vi "Begin.vi"() -> (0 "error out":errorcluster)   [LabVIEW 2012]
doc: "Called before other user functions, this VI is expected to open initial I/O refnums, load in file data, and do all program initialization. Notice that the <B>error out</B> terminal is simply used for data flow. Wiring it to other structures or subVIs ensures that this VI runs first."
uses:
  <vilib>/Rock Robotics/WPI/Joystick/WPI_JoystickDeviceEnum.ctl
  <vilib>/Rock Robotics/SystemInterfaces/Typedef/FPGA_TypedefDigitalModule.ctl
  <vilib>/Rock Robotics/SystemInterfaces/DIO/FPGA_DIOPWMChannel.ctl
  <vilib>/Rock Robotics/WPI/SafetyOutput/WPI_SafetyOutputConfigMenu.ctl
  <vilib>/Rock Robotics/WPI/CAN/Jaguar/SubVIs/WPI_CANJaguar_ControlMode.ctl
  <vilib>/Rock Robotics/WPI/CAN/Jaguar/SubVIs/WPI_CANJaguar_SpeedReference.ctl
  <vilib>/Rock Robotics/WPI/CAN/Jaguar/SubVIs/WPI_CANJaguar_BrakeCoastMode.ctl
  Robot Global Data.vi
  <vilib>/Rock Robotics/WPI/MotorControl/WPI_MotorControlOpen Victor.vi
  <vilib>/Rock Robotics/WPI/MotorControl/WPI_MotorControlOpenCANJaguar.vi
  <vilib>/Rock Robotics/WPI/RobotDrive/WPI_RobotDriveOpen2MotorWithCANJaguar.vi
  <vilib>/Rock Robotics/SystemInterfaces/AI/FPGA_AIGyroChannel.ctl
  <vilib>/Rock Robotics/SystemInterfaces/Typedef/FPGA_TypedefAnalogModuleForGyro.ctl
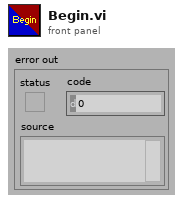
[diagram p1: front panel]
types:
  T1 = typedef "WPI_SafetyOutputConfigMenu.ctl" = enum16{"Enable", "Disable"}
  T2 = typedef "FPGA_DIOPWMChannel.ctl" = enum8{"PWM 1", "PWM 2", "PWM 3", "PWM 4", "PWM 5", "PWM 6", "PWM 7", "PWM 8", "PWM 9", "PWM 10", "Invalid"}
  T3 = typedef "FPGA_TypedefDigitalModule.ctl" = enum16{"Digital Module 1", "Digital Module 2"}
  T4 = typedef "WPI_JoystickDeviceEnum.ctl" = enum16{"USB 1", "USB 2", "USB 3", "USB 4", "Kinect 1", "Kinect 2"}
  T5 = typedef "WPI_MotorControlDeviceRef.ctl" = cluster{"DeviceStatus":errorcluster, "Type":enum16{"PWM", "CAN"}, "PWM":cluster{"Digital Module":T3, "PWM Channel":T2, "DeadBand":T6}, "CAN":cluster{"Device Number":u8, "Control Mode":T7, "Semaphore":T8, "Max Vout":dbl}, "Invert":bool, "TransformRef":T9, "InvTransformRef":T9}
  T6 = typedef "WPI_PWMDeadband.ctl" = cluster{"Name":string, "maxPositivePwm":i32, "minPositivePwm":i32, "centerPwm":i32, "maxNegativePwm":i32, "minNegativePwm":i32, "angularRange":u16}
  T7 = typedef "WPI_CANJaguar_ControlMode.ctl" = enum8{"Percent VBus", "Current", "Speed", "Position", "Voltage"}
  T8 = typedef "Semaphore RefNum" = refnum<k1>
  T9 = typedef "WPI_PWMTransform_ConPane.ctl" = refnum<vi>
  T10 = typedef "WPI_ServoDeviceRef.ctl" = cluster{"DeviceStatus":errorcluster, "Digital Module":T3, "PWM Channel":T2, "DeadBand":T6}
  T11 = typedef "WPI_RobotDriveDevRef.ctl" = cluster{"DevStatus":errorcluster, "Motors[]":T5[], "Square Inputs":bool, "Max Output":dbl, "Isochronous":bool}
  T12 = typedef "WPI_CANJaguar_BrakeCoastMode.ctl" = enum8{"Jumper", "Brake", "Coast"}
  T13 = typedef "WPI_CANJaguar_SpeedReference.ctl" = u8
  T14 = typedef "WPI_JoystickDevRef.ctl" = cluster{"Device":T4}
  T15 = typedef "FPGA_TypedefAnalogModuleForGyro.ctl" = enum16{"Analog Module 1"}
  T16 = typedef "FPGA_AIGyroChannel.ctl" = enum8{"AI 1", "AI 2", "Invalid"}
  T17 = typedef "WPI_GyroDevRef.ctl" = cluster{"DevStatus":errorcluster, "Analog Module":T18, "Analog Channel":T19, "Offset":dbl, "Gain (VoltsPerDegree/Second)":dbl}
  T18 = typedef "FPGA_TypedefAnalogModule.ctl" = enum16{"Analog Module 1", "Analog Module 2"}
  T19 = typedef "FPGA_AIChannel.ctl" = enum8{"AI 1", "AI 2", "AI 3", "AI 4", "AI 5", "AI 6", "AI 7", "AI 8", "Invalid"}
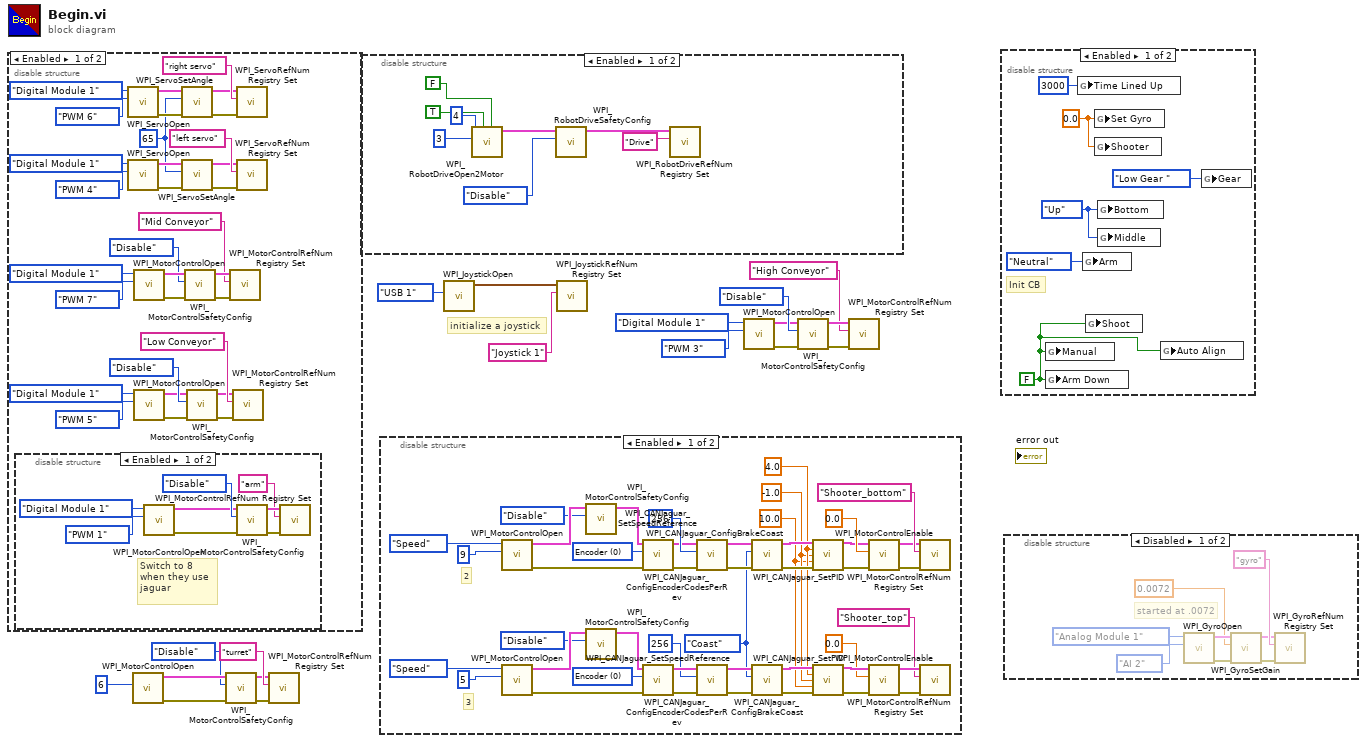
[diagram p0: block diagram]
diagram:
  # "initialize a joystick"
  n1 = disable-structure shown="Enabled" {
    frame Enabled {
      w19 = 65 ("Angle")
      n2 = disable-structure shown="Enabled" {
        frame Enabled {
          # "Switch to 8\nwhen they use\njaguar"
          n3 = call-poly <vilib>:"WPI_MotorControlOpen.vi"("PWM Channel"=FPGA_DIOPWMChannel."PWM 1", "Digital Module (Module 1)"=FPGA_TypedefDigitalModule."Digital Module 1") -> ("error out"=w53:errorcluster, "MotorControlDeviceRef"=w54:T5)  [unwired: 8 in]
          n4 = call <vilib>:"WPI_MotorControlSafetyConfig.vi"("error in (no error)"=w53, "mode"=WPI_SafetyOutputConfigMenu."Disable", "MotorControlDevRef"=w54) -> ("error out"=w51:errorcluster, "MotorControlDevRef"=w52:T5)  [unwired: 7 in]
          n5 = call <vilib>:"WPI_MotorControlRefNum Registry Set.vi"("error in (no error)"=w51, "refnum name"="arm", "MotorControlDevRef"=w52) -> ()  [unwired: 7 in, 2 out]
        }
        frame Disabled {
        }
      }
      n6 = call <vilib>:"WPI_ServoOpen.vi"("PWM Channel"=FPGA_DIOPWMChannel."PWM 6", "Digital Module (Module 1)"=FPGA_TypedefDigitalModule."Digital Module 1") -> ("error out"=w25:errorcluster, "ServoDeviceRef"=w27:T10)  [unwired: 8 in]
      n7 = call <vilib>:"WPI_ServoOpen.vi"("PWM Channel"=FPGA_DIOPWMChannel."PWM 4", "Digital Module (Module 1)"=FPGA_TypedefDigitalModule."Digital Module 1") -> ("error out"=w21:errorcluster, "ServoDeviceRef"=w23:T10)  [unwired: 8 in]
      n8 = call-poly <vilib>:"WPI_MotorControlOpen.vi"("PWM Channel"=FPGA_DIOPWMChannel."PWM 7", "Digital Module (Module 1)"=FPGA_TypedefDigitalModule."Digital Module 1") -> ("error out"=w41:errorcluster, "MotorControlDeviceRef"=w40:T5)  [unwired: 8 in]
      n9 = call-poly <vilib>:"WPI_MotorControlOpen.vi"("PWM Channel"=FPGA_DIOPWMChannel."PWM 5", "Digital Module (Module 1)"=FPGA_TypedefDigitalModule."Digital Module 1") -> ("error out"=w31:errorcluster, "MotorControlDeviceRef"=w32:T5)  [unwired: 8 in]
      n10 = call <vilib>:"WPI_ServoSetAngle.vi"("error in (no error)"=w25, "Angle"=w19, "ServoDeviceRef"=w27) -> ("error out"=w24:errorcluster, "ServoDeviceRef"=w26:T10)  [unwired: 7 in]
      n11 = call <vilib>:"WPI_ServoSetAngle.vi"("error in (no error)"=w21, "Angle"=w19, "ServoDeviceRef"=w23) -> ("error out"=w20:errorcluster, "ServoDeviceRef"=w22:T10)  [unwired: 7 in]
      n12 = call <vilib>:"WPI_MotorControlSafetyConfig.vi"("error in (no error)"=w41, "mode"=WPI_SafetyOutputConfigMenu."Disable", "MotorControlDevRef"=w40) -> ("error out"=w43:errorcluster, "MotorControlDevRef"=w42:T5)  [unwired: 7 in]
      n13 = call <vilib>:"WPI_MotorControlSafetyConfig.vi"("error in (no error)"=w31, "mode"=WPI_SafetyOutputConfigMenu."Disable", "MotorControlDevRef"=w32) -> ("error out"=w29:errorcluster, "MotorControlDevRef"=w30:T5)  [unwired: 7 in]
      n14 = call <vilib>:"WPI_MotorControlRefNum Registry Set.vi"("error in (no error)"=w43, "refnum name"="Mid Conveyor", "MotorControlDevRef"=w42) -> ()  [unwired: 7 in, 2 out]
      n15 = call <vilib>:"WPI_MotorControlRefNum Registry Set.vi"("error in (no error)"=w29, "refnum name"="Low Conveyor", "MotorControlDevRef"=w30) -> ()  [unwired: 7 in, 2 out]
      n16 = call <vilib>:"WPI_ServoRefNum Registry Set.vi"("error in (no error)"=w24, "refnum name"="right servo", "ServoDeviceRef"=w26) -> ()  [unwired: 7 in, 2 out]
      n17 = call <vilib>:"WPI_ServoRefNum Registry Set.vi"("error in (no error)"=w20, "refnum name"="left servo", "ServoDeviceRef"=w22) -> ()  [unwired: 7 in, 2 out]
    }
    frame Disabled {
    }
  }
  n18 = call-poly <vilib>:"WPI_MotorControlOpen.vi"("Device Number"=u8 6) -> ("error out"=w4:errorcluster, "MotorControlDeviceRef"=w3:T5)  [unwired: 9 in]
  n19 = call <vilib>:"WPI_MotorControlSafetyConfig.vi"("error in (no error)"=w4, "mode"=WPI_SafetyOutputConfigMenu."Disable", "MotorControlDevRef"=w3) -> ("error out"=w6:errorcluster, "MotorControlDevRef"=w5:T5)  [unwired: 7 in]
  n20 = call <vilib>:"WPI_MotorControlRefNum Registry Set.vi"("error in (no error)"=w6, "refnum name"="turret", "MotorControlDevRef"=w5) -> ()  [unwired: 7 in, 2 out]
  n21 = disable-structure shown="Enabled" {
    frame Enabled {
      n22 = call-poly <vilib>:"WPI_RobotDriveOpen2Motor.vi"("Right Motor Inverted"=FALSE, "Left Motor Inverted"=TRUE, "Right Motor"=u8 3, "Left Motor"=u8 4) -> ("RobotDriveDevRef"=w62:T11)  [unwired: 6 in, 1 out]
      n23 = call <vilib>:"WPI_RobotDriveSafetyConfig.vi"("mode"=WPI_SafetyOutputConfigMenu."Disable", "RobotDriveDevRef"=w62) -> ("RobotDriveDevRef"=w61:T11)  [unwired: 8 in, 1 out]
      n24 = call <vilib>:"WPI_RobotDriveRefNum Registry Set.vi"("refnum name"="Drive", "RobotDriveDevRef"=w61) -> ()  [unwired: 8 in, 2 out]
    }
    frame Disabled {
    }
  }
  n25 = disable-structure shown="Enabled" {
    frame Enabled {
      w75 = WPI_CANJaguar_BrakeCoastMode."Coast" ("Brake / Coast Mode")
      w66 = 10.0 ("D")
      w67 = -1.0 ("I")
      w68 = 4.0 ("P")
      w87 = T13 0 items=["Encoder"=0, "Inv Encoder"=2, "Quad Encoder"=3, "None"=255] ("Speed Reference")
      w104 = T13 0 items=["Encoder"=0, "Inv Encoder"=2, "Quad Encoder"=3, "None"=255] ("Speed Reference")
      # "2"
      # "3"
      n26 = call-poly <vilib>:"WPI_MotorControlOpen.vi"("Device Number"=u8 9, "Control Mode"=WPI_CANJaguar_ControlMode."Speed") -> ("error out"=w86:errorcluster, "MotorControlDeviceRef"=w85:T5)  [unwired: 8 in]
      n27 = call-poly <vilib>:"WPI_MotorControlOpen.vi"("Device Number"=u8 5, "Control Mode"=WPI_CANJaguar_ControlMode."Speed") -> ("error out"=w105:errorcluster, "MotorControlDeviceRef"=w106:T5)  [unwired: 8 in]
      n28 = call <vilib>:"WPI_MotorControlSafetyConfig.vi"("mode"=WPI_SafetyOutputConfigMenu."Disable", "MotorControlDevRef"=w85) -> ("MotorControlDevRef"=w72:T5)  [unwired: 8 in, 1 out]
      n29 = call <vilib>:"WPI_MotorControlSafetyConfig.vi"("mode"=WPI_SafetyOutputConfigMenu."Disable", "MotorControlDevRef"=w106) -> ("MotorControlDevRef"=w70:T5)  [unwired: 8 in, 1 out]
      n30 = call <vilib>:"WPI_CANJaguar_SetSpeedReference.vi"("error in (no error)"=w86, "Speed Reference"=w87, "CAN Jaguar Ref"=w72) -> ("error out"=w89:errorcluster, "CAN Jaguar Ref Out"=w84:T5)  [unwired: 7 in]
      n31 = call <vilib>:"WPI_CANJaguar_SetSpeedReference.vi"("error in (no error)"=w105, "Speed Reference"=w104, "CAN Jaguar Ref"=w70) -> ("error out"=w102:errorcluster, "CAN Jaguar Ref Out"=w107:T5)  [unwired: 7 in]
      n32 = call <vilib>:"WPI_CANJaguar_ConfigEncoderCodesPerRev.vi"("error in (no error)"=w89, "Encoder Codes Per Rev"=u16 256, "CAN Jaguar Ref"=w84) -> ("error out"=w76:errorcluster, "CAN Jaguar Ref Out"=w77:T5)  [unwired: 7 in]
      n33 = call <vilib>:"WPI_CANJaguar_ConfigEncoderCodesPerRev.vi"("error in (no error)"=w102, "Encoder Codes Per Rev"=u16 256, "CAN Jaguar Ref"=w107) -> ("error out"=w80:errorcluster, "CAN Jaguar Ref Out"=w81:T5)  [unwired: 7 in]
      n34 = call <vilib>:"WPI_CANJaguar_ConfigBrakeCoast.vi"("error in (no error)"=w76, "Brake / Coast Mode"=w75, "CAN Jaguar Ref"=w77) -> ("error out"=w73:errorcluster, "CAN Jaguar Ref Out"=w74:T5)  [unwired: 7 in]
      n35 = call <vilib>:"WPI_CANJaguar_ConfigBrakeCoast.vi"("error in (no error)"=w80, "Brake / Coast Mode"=w75, "CAN Jaguar Ref"=w81) -> ("error out"=w78:errorcluster, "CAN Jaguar Ref Out"=w79:T5)  [unwired: 7 in]
      n36 = call <vilib>:"WPI_CANJaguar_SetPID.vi"("CAN Jaguar Ref"=w74, "P"=w68, "I"=w67, "D"=w66, "error in (no error)"=w73) -> ("CAN Jaguar Ref Out"=w90:T5, "error out"=w91:errorcluster)  [unwired: 9 in]
      n37 = call <vilib>:"WPI_CANJaguar_SetPID.vi"("CAN Jaguar Ref"=w79, "P"=w68, "I"=w67, "D"=w66, "error in (no error)"=w78) -> ("CAN Jaguar Ref Out"=w101:T5, "error out"=w100:errorcluster)  [unwired: 9 in]
      n38 = call <vilib>:"WPI_MotorControlEnable.vi"("error in (no error)"=w91, "Encoder Initial Position"=0.0, "CAN Jaguar Ref"=w90) -> ("error out"=w94:errorcluster, "CAN Jaguar Ref Out"=w93:T5)  [unwired: 7 in]
      n39 = call <vilib>:"WPI_MotorControlEnable.vi"("error in (no error)"=w100, "Encoder Initial Position"=0.0, "CAN Jaguar Ref"=w101) -> ("error out"=w97:errorcluster, "CAN Jaguar Ref Out"=w98:T5)  [unwired: 7 in]
      n40 = call <vilib>:"WPI_MotorControlRefNum Registry Set.vi"("error in (no error)"=w94, "refnum name"="Shooter_bottom", "MotorControlDevRef"=w93) -> ()  [unwired: 7 in, 2 out]
      n41 = call <vilib>:"WPI_MotorControlRefNum Registry Set.vi"("error in (no error)"=w97, "refnum name"="Shooter_top", "MotorControlDevRef"=w98) -> ()  [unwired: 7 in, 2 out]
    }
    frame Disabled {
    }
  }
  n42 = call <vilib>:"WPI_JoystickOpen.vi"("JoystickDevice"=WPI_JoystickDeviceEnum."USB 1") -> ("JoystickDevRef"=w18:T14)  [unwired: 10 out]
  n43 = call <vilib>:"WPI_JoystickRefNum Registry Set.vi"("refnum name"="Joystick 1", "JoystickDevRef"=w18) -> ()  [unwired: 1 in, 9 out]
  n44 = call-poly <vilib>:"WPI_MotorControlOpen.vi"("PWM Channel"=FPGA_DIOPWMChannel."PWM 3", "Digital Module (Module 1)"=FPGA_TypedefDigitalModule."Digital Module 1") -> ("error out"=w12:errorcluster, "MotorControlDeviceRef"=w11:T5)  [unwired: 8 in]
  n45 = call <vilib>:"WPI_MotorControlSafetyConfig.vi"("error in (no error)"=w12, "mode"=WPI_SafetyOutputConfigMenu."Disable", "MotorControlDevRef"=w11) -> ("error out"=w14:errorcluster, "MotorControlDevRef"=w13:T5)  [unwired: 7 in]
  n46 = call <vilib>:"WPI_MotorControlRefNum Registry Set.vi"("error in (no error)"=w14, "refnum name"="High Conveyor", "MotorControlDevRef"=w13) -> ()  [unwired: 7 in, 2 out]
  n47 = disable-structure shown="Enabled" {
    frame Enabled {
      w112 = 0.0 ("Shooter")
      w110 = FALSE ("Shoot")
      w115 = enum16{"Up", "Neutral", "Down"}."Up" ("Top")
      # "Init CB"
      n48 = global write "Robot Global Data.vi" "Manual"(w110) -> ()
      n49 = global write "Robot Global Data.vi" "Arm Down"(w110) -> ()
      n50 = global write "Robot Global Data.vi" "Time Lined Up"(3000 ("Time Lined Up")) -> ()
      n51 = global write "Robot Global Data.vi" "Arm"(enum16{"Up", "Neutral", "Down"}."Neutral" ("Top")) -> ()
      n52 = global write "Robot Global Data.vi" "Shoot"(w110) -> ()
      n53 = global write "Robot Global Data.vi" "Set Gyro"(w112) -> ()
      n54 = global write "Robot Global Data.vi" "Shooter"(w112) -> ()
      n55 = global write "Robot Global Data.vi" "Bottom"(w115) -> ()
      n56 = global write "Robot Global Data.vi" "Middle"(w115) -> ()
      n57 = global write "Robot Global Data.vi" "Auto Align"(w110) -> ()
      n58 = global write "Robot Global Data.vi" "Gear"(enum16{"Low Gear ", "None", "High Gear"}."Low Gear " ("Gear")) -> ()
    }
    frame Disabled {
    }
  }
  n59 = disable-structure shown="Disabled" {
    frame Disabled {
      # "started at .0072"
      n60 = call <vilib>:"WPI_GyroOpen.vi"("Analog Channel"=FPGA_AIGyroChannel."AI 2", "Analog Module (Module 1)"=FPGA_TypedefAnalogModuleForGyro."Analog Module 1") -> ("error out"=w117:errorcluster, "GyroDevRef"=w118:T17)  [unwired: 7 in, 1 out]
      n61 = call <vilib>:"WPI_GyroSetGain.vi"("error in (no error)"=w117, "Gain (VoltsPerDegree/Second)"=0.0072, "GyroDevRef"=w118) -> ("error out"=w120:errorcluster, "GyroDevRef"=w119:T17)  [unwired: 7 in]
      n62 = call <vilib>:"WPI_GyroRefNum Registry Set.vi"("error in (no error)"=w120, "refnum name"="gyro", "GyroDevRef"=w119) -> ()  [unwired: 7 in, 2 out]
    }
    frame Enabled {
    }
  }
